vi "gyro-fitter-V1.vi"() -> ()   [LabVIEW 2018]
uses:
  plot refs -- filter related.ctl
  cursor window action.ctl
  publisher action.ctl
  circle corners.ctl
  lorentzian.ctl
  peak -- parameters -- complex fit.ctl
  wavepacket.ctl
  filter method control.ctl
  parameters -- scan monitor control.ctl
panel:
  in  "Tab :  Fit controls":T1(tab)
  out "lorentzian":T2={"A (VHz)"=1.3498083421914207e-06, "f (Hz)"=20818.316775416508, "G (Hz)"=65.7151812568016, "phi(rad)"=4.172856066514944, "Q"=316.7961554281156, "Norm  Ampl"=nan, "bg (V)"=-2.924526385728085e-08-2.2207879205523747e-08i, "4corners"={"z (-pi/2)"=-5.7420040702404924e-08-2.9278119892568764e-08i, "z(inf)"=-2.924526385728085e-08-2.2207879205523747e-08i, "z (pi/2)"=-3.6315504544325864e-08+5.9668976396003224e-09i, "z center"=-4.6867772623365394e-08-1.1655611126484221e-08i, "z(0)"=-6.449028138944994e-08-1.1033430474446945e-09i, "radius"=2.0540281809718265e-08}} {"bg (V)" format="%#9_9f"; "Q" format="%#9_9f"; "phi(rad)" format="%#9_9f"; "G (Hz)" format="%#9_9f"; "f (Hz)" format="%#9_9f"}
  in  "Plot: fragment - filter":cluster{dbl[], dbl[]}[](graph)=[{array[248 elements], array[248 elements]}, {array[248 elements], array[248 elements]}, {array[248 elements], array[248 elements]}, {array[248 elements], array[248 elements]}]
  out "Plot: phase around center":cluster{dbl[], dbl[]}[](graph)
  out "Plot: fragment":cluster{dbl[], dbl[]}[](graph)
  out "Plot: complex plane":cluster{dbl[], dbl[]}[](graph)=[{array[248 elements], array[248 elements]}, {[-2.632749081364713e-08, -2.6489457070801555e-08, -2.6972801537635557e-08, -2.7769901583171174e-08, -2.886818646352582e-08, -3.025033557005272e-08, -3.189455158568609e-08, -3.3774904241652344e-08, -3.586173925329867e-08, -3.81221459858766e-08, -4.0520476474911847e-08, -4.301890761589914e-08, -4.557803765725468e-08, -4.815750758947611e-08, -5.0716637630831656e-08, -5.321506877181894e-08, -5.561339926085419e-08, -5.7873805993432123e-08, -5.996064100507845e-08, -6.184099366104471e-08, -6.348520967667807e-08, -6.486735878320497e-08, -6.596564366355961e-08, -6.676274370909523e-08, -6.724608817592924e-08, -6.740805443308366e-08, -6.724608817592924e-08, -6.676274370909523e-08, -6.596564366355961e-08, -6.486735878320496e-08, -6.348520967667807e-08, -6.18409936610447e-08, -5.996064100507845e-08, -5.787380599343211e-08, -5.5613399260854173e-08, -5.321506877181894e-08, -5.071663763083165e-08, -4.815750758947611e-08, -4.5578037657254674e-08, -4.3018907615899126e-08, -4.052047647491185e-08, -3.81221459858766e-08, -3.586173925329867e-08, -3.377490424165234e-08, -3.1894551585686074e-08, -3.025033557005271e-08, -2.886818646352582e-08, -2.776990158317117e-08, -2.6972801537635557e-08, -2.6489457070801555e-08], [-1.1655611126484221e-08, -9.081231188950172e-09, -6.547450760891066e-09, -4.0942290732644576e-09, -1.7602548975678168e-09, 4.176635991995252e-10, 2.4051793413181066e-09, 4.1709480182503586e-09, 5.687122403141979e-09, 6.929791520224554e-09, 7.879357735187145e-09, 8.520845821576428e-09, 8.844139129063635e-09, 8.844139129063635e-09, 8.520845821576428e-09, 7.879357735187142e-09, 6.929791520224554e-09, 5.687122403141975e-09, 4.170948018250355e-09, 2.4051793413181033e-09, 4.1766359919952687e-10, -1.7602548975678184e-09, -4.0942290732644625e-09, -6.547450760891066e-09, -9.081231188950175e-09, -1.1655611126484228e-08, -1.4229991064018272e-08, -1.676377149207738e-08, -1.9216993179703993e-08, -2.1550967355400627e-08, -2.3728885852167972e-08, -2.5716401594286547e-08, -2.74821702712188e-08, -2.8998344656110424e-08, -3.0241013773193e-08, -3.1190579988155584e-08, -3.183206807454487e-08, -3.215536138203208e-08, -3.215536138203208e-08, -3.183206807454487e-08, -3.1190579988155584e-08, -3.0241013773192996e-08, -2.8998344656110417e-08, -2.7482170271218794e-08, -2.571640159428654e-08, -2.372888585216796e-08, -2.1550967355400623e-08, -1.9216993179703983e-08, -1.676377149207737e-08, -1.422999106401826e-08]}, {[-2.924526385728085e-08, -3.10075147338893e-08, -3.276976561049776e-08, -3.4532016487106214e-08, -3.629426736371467e-08, -3.805651824032312e-08, -3.981876911693158e-08, -4.158101999354003e-08, -4.334327087014848e-08, -4.510552174675694e-08, -4.6867772623365394e-08, -4.8630023499973846e-08, -5.0392274376582305e-08, -5.215452525319076e-08, -5.391677612979921e-08, -5.567902700640767e-08, -5.744127788301612e-08, -5.9203528759624574e-08, -6.096577963623303e-08, -6.272803051284148e-08], [-2.2207879205523747e-08, -2.1152652397619794e-08, -2.0097425589715843e-08, -1.904219878181189e-08, -1.7986971973907936e-08, -1.6931745166003982e-08, -1.5876518358100032e-08, -1.4821291550196078e-08, -1.3766064742292127e-08, -1.2710837934388175e-08, -1.1655611126484221e-08, -1.0600384318580269e-08, -9.545157510676317e-09, -8.489930702772363e-09, -7.434703894868411e-09, -6.379477086964459e-09, -5.324250279060506e-09, -4.269023471156552e-09, -3.2137966632526018e-09, -2.158569855348648e-09]}, {[-5.7420040702404924e-08, -5.636481389450097e-08, -5.5309587086597017e-08, -5.425436027869306e-08, -5.319913347078911e-08, -5.214390666288516e-08, -5.10886798549812e-08, -5.0033453047077255e-08, -4.89782262391733e-08, -4.792299943126935e-08, -4.6867772623365394e-08, -4.581254581546144e-08, -4.475731900755749e-08, -4.370209219965353e-08, -4.264686539174958e-08, -4.1591638583845626e-08, -4.053641177594168e-08, -3.948118496803772e-08, -3.842595816013377e-08, -3.737073135222982e-08], [-2.9278119892568764e-08, -2.751586901596031e-08, -2.5753618139351856e-08, -2.39913672627434e-08, -2.2229116386134948e-08, -2.0466865509526493e-08, -1.8704614632918037e-08, -1.6942363756309585e-08, -1.518011287970113e-08, -1.3417862003092673e-08, -1.1655611126484221e-08, -9.893360249875765e-09, -8.13110937326731e-09, -6.368858496658857e-09, -4.606607620050402e-09, -2.8443567434419492e-09, -1.0821058668334936e-09, 6.801450097749588e-10, 2.4423958863834177e-09, 4.20464676299187e-09]}, {[-0.03712059630022613, -0.04038900428695615, -0.043632170488046795, -0.04684806803019193, -0.050034687082109765, -0.053190036110621716, -0.05631214312529604, -0.05939905691087754, -0.06244884824673365, -0.06545961111255436, -0.06842946387955313, -0.07135655048642349, -0.07423904159931691, -0.07707513575511701, -0.07986306048729519, -0.08260107343364476, -0.08528746342520038, -0.08792055155566313, -0.09049869223066223, -0.09302027419619781], [0.13121393299301523, 0.1302450136134994, 0.12919469531706476, 0.12806363451845718, 0.1268525380938582, 0.12556216293911035, 0.12419331549668176, 0.12274685125166607, 0.12122367419713193, 0.11962473626915691, 0.11795103675189833, 0.11620362165307317, 0.11438358305023741, 0.11249205840827295, 0.11053022986850931, 0.10849932350992353, 0.10640060858288088, 0.10423539671589463, 0.10200504109590092, 0.09971093562256111]}, {[-0.0412038570844881, -0.04483178994975843, -0.04843170443296904, -0.05200135070475014, -0.05553849785237894, -0.059040935274027206, -0.0625064740603157, -0.06593294836231116, -0.06931821674511145, -0.07266016352617244, -0.07595670009754107, -0.07920576623116717, -0.08240533136647886, -0.08555339587941699, -0.08864799233213477, -0.09168718670258277, -0.09466907959320953, -0.09759180741802317, -0.10045354356727218, -0.10325249954901668], [0.14564746968253484, 0.1445719691712723, 0.14340611586222982, 0.1421506383757754, 0.14080632134447055, 0.1393740049227004, 0.13785458426160468, 0.13624900894963726, 0.13455828241910436, 0.13278346131905208, 0.13092565485489507, 0.12898602409519913, 0.12696578124605143, 0.12486618889347091, 0.12268855921433326, 0.12043425315630304, 0.11810467958728571, 0.11570129441493096, 0.11322559967673795, 0.11067914260133077]}, {array[248 elements], array[248 elements]}]
  in  "scale gauge: Plot: complex plane":dbl(slide)=0.00275 min=0.0 max=0.3 step=1e-06 scale=1e-05..0.5 scale format="%#_3p"
  out "Plot: phase":cluster{"omega out":dbl[], dbl[]}(graph)
  out "Plot: win omega":T4(graph)
  out "Plot: dz/domega":cluster{"omega out":dbl[], dbl[]}(graph)
  in  "Plot: complex plane - filter":cluster{dbl[], dbl[]}[](graph)=[{array[248 elements], array[248 elements]}, {array[248 elements], array[248 elements]}, {[1.0007727048625014e-06, 9.989970596885263e-07, 9.936771318268878e-07, 9.848339166024118e-07, 9.725023141455088e-07, 9.567309916573026e-07, 9.375821913424224e-07, 9.151314847674563e-07, 8.894674746145036e-07, 8.606914450068672e-07, 8.289169617868905e-07, 7.942694243234624e-07, 7.568855706179972e-07, 7.169129376620118e-07, 6.745092791760248e-07, 6.298419430276915e-07, 5.830872107862246e-07, 5.344296020195755e-07, 4.840611460799999e-07, 4.3218062425193193e-07, 3.7899278525307166e-07, 3.247075371847349e-07, 2.6953911912047683e-07, 2.1370525560234447e-07, 1.574262973815776e-07, 1.0092435179486355e-07, 4.4422406208149694e-08, -1.1856552012617152e-08, -6.76904155307497e-08, -1.228588335950076e-07, -1.7714408166334431e-07, -2.303319206622046e-07, -2.822124424902725e-07, -3.325808984298484e-07, -3.812385071964974e-07, -4.2799323943796406e-07, -4.726605755862975e-07, -5.150642340722845e-07, -5.550368670282699e-07, -5.924207207337353e-07, -6.27068258197163e-07, -6.588427414171397e-07, -6.876187710247764e-07, -7.13282781177729e-07, -7.357334877526951e-07, -7.548822880675753e-07, -7.706536105557815e-07, -7.829852130126845e-07, -7.918284282371605e-07, -7.97148356098799e-07, -7.989240012727741e-07, -7.97148356098799e-07, -7.918284282371605e-07, -7.829852130126845e-07, -7.706536105557813e-07, -7.548822880675751e-07, -7.357334877526949e-07, -7.13282781177729e-07, -6.876187710247761e-07, -6.588427414171397e-07, -6.27068258197163e-07, -5.924207207337349e-07, -5.550368670282699e-07, -5.150642340722845e-07, -4.726605755862974e-07, -4.2799323943796427e-07, -3.8123850719649685e-07, -3.3258089842984826e-07, -2.82212442490272e-07, -2.3033192066220443e-07, -1.7714408166334437e-07, -1.2285883359500722e-07, -6.769041553074954e-08, -1.185655201261657e-08, 4.442240620814987e-08, 1.0092435179486354e-07, 1.5742629738157798e-07, 2.1370525560234442e-07, 2.6953911912047736e-07, 3.247075371847351e-07, 3.7899278525307145e-07, 4.3218062425193225e-07, 4.840611460799998e-07, 5.344296020195761e-07, 5.830872107862246e-07, 6.298419430276921e-07, 6.74509279176025e-07, 7.169129376620118e-07, 7.568855706179976e-07, 7.942694243234626e-07, 8.289169617868909e-07, 8.606914450068672e-07, 8.894674746145036e-07, 9.151314847674565e-07, 9.375821913424224e-07, 9.567309916573028e-07, 9.725023141455088e-07, 9.848339166024118e-07, 9.93677131826888e-07, 9.989970596885263e-07], [-7.941413356603459e-08, -2.2912187979320604e-08, 3.336677024144617e-08, 8.920063375957865e-08, 1.4436905182383665e-07, 1.9865429989217332e-07, 2.518421388910337e-07, 3.0372266071910163e-07, 3.5409111665867737e-07, 4.027487254253263e-07, 4.4950345766679327e-07, 4.941707938151267e-07, 5.365744523011137e-07, 5.76547085257099e-07, 6.139309389625643e-07, 6.485784764259922e-07, 6.803529596459688e-07, 7.091289892536055e-07, 7.347929994065581e-07, 7.572437059815242e-07, 7.763925062964043e-07, 7.921638287846105e-07, 8.044954312415137e-07, 8.133386464659896e-07, 8.186585743276281e-07, 8.204342195016031e-07, 8.186585743276281e-07, 8.133386464659896e-07, 8.044954312415136e-07, 7.921638287846105e-07, 7.763925062964043e-07, 7.572437059815242e-07, 7.347929994065581e-07, 7.091289892536053e-07, 6.803529596459686e-07, 6.485784764259922e-07, 6.139309389625643e-07, 5.765470852570989e-07, 5.365744523011135e-07, 4.941707938151265e-07, 4.495034576667934e-07, 4.027487254253263e-07, 3.540911166586773e-07, 3.037226607191014e-07, 2.518421388910335e-07, 1.9865429989217305e-07, 1.4436905182383667e-07, 8.920063375957859e-08, 3.3366770241446023e-08, -2.2912187979320816e-08, -7.941413356603488e-08, -1.3591607915274855e-07, -1.921950373735154e-07, -2.4802890089164793e-07, -3.0319731895590604e-07, -3.5748256702424276e-07, -4.106704060231032e-07, -4.6255092785117075e-07, -5.129193837907467e-07, -5.615769925573957e-07, -6.083317247988627e-07, -6.529990609471961e-07, -6.954027194331829e-07, -7.353753523891683e-07, -7.727592060946336e-07, -8.074067435580613e-07, -8.391812267780381e-07, -8.679572563856746e-07, -8.936212665386275e-07, -9.160719731135933e-07, -9.352207734284734e-07, -9.509920959166797e-07, -9.633236983735828e-07, -9.72166913598059e-07, -9.774868414596972e-07, -9.792624866336723e-07, -9.774868414596972e-07, -9.721669135980588e-07, -9.633236983735828e-07, -9.509920959166796e-07, -9.352207734284736e-07, -9.160719731135932e-07, -8.936212665386273e-07, -8.679572563856744e-07, -8.391812267780379e-07, -8.07406743558061e-07, -7.727592060946332e-07, -7.353753523891682e-07, -6.954027194331825e-07, -6.529990609471957e-07, -6.083317247988619e-07, -5.615769925573952e-07, -5.129193837907467e-07, -4.6255092785117033e-07, -4.1067040602310277e-07, -3.574825670242419e-07, -3.0319731895590556e-07, -2.480289008916479e-07, -1.921950373735149e-07, -1.3591607915274848e-07]}, {[8.158298491348722e-07, 1.4464037823280978e-07, -1.4742601783239322e-07], [2.2455224868565569e-07, -4.250242519508206e-08, -2.2568975850353674e-07]}, {[1.4646634674448616e-08, 5.3243073422403955e-09, -3.998019989967825e-09, -1.3320347322176047e-08, -2.2642674654384265e-08, -3.1965001986592484e-08, -4.128732931880071e-08, -5.060965665100893e-08, -5.993198398321715e-08, -6.925431131542536e-08, -7.857663864763358e-08, -8.78989659798418e-08, -9.722129331205003e-08, -1.0654362064425824e-07, -1.1586594797646647e-07, -1.2518827530867468e-07, -1.345106026408829e-07, -1.4383292997309114e-07, -1.5315525730529934e-07, -1.6247758463750758e-07], [3.0693237684966145e-08, 2.3232631101344026e-08, 1.5772024517721908e-08, 8.31141793409979e-09, 8.508113504776711e-10, -6.609795233144444e-09, -1.4070401816766566e-08, -2.1531008400388688e-08, -2.8991614984010803e-08, -3.645222156763292e-08, -4.391282815125503e-08, -5.137343473487716e-08, -5.8834041318499277e-08, -6.629464790212139e-08, -7.375525448574352e-08, -8.121586106936564e-08, -8.867646765298775e-08, -9.613707423660988e-08, -1.0359768082023198e-07, -1.1105828740385411e-07]}, {[1.4464037823280976e-07, 1.5714332117450805e-07, 1.6964626411620634e-07, 1.8214920705790464e-07, 1.9465214999960293e-07, 2.0715509294130122e-07, 2.1965803588299952e-07, 2.321609788246978e-07, 2.446639217663961e-07, 2.5716686470809437e-07, 2.696698076497927e-07, 2.82172750591491e-07, 2.946756935331893e-07, 3.0717863647488754e-07, 3.1968157941658586e-07, 3.321845223582842e-07, 3.4468746529998245e-07, 3.571904082416807e-07, 3.6969335118337904e-07, 3.8219629412507736e-07], [-4.250242519508206e-08, -4.250242519508206e-08, -4.250242519508206e-08, -4.250242519508206e-08, -4.250242519508206e-08, -4.250242519508206e-08, -4.250242519508206e-08, -4.250242519508206e-08, -4.250242519508206e-08, -4.250242519508206e-08, -4.250242519508206e-08, -4.250242519508206e-08, -4.250242519508206e-08, -4.250242519508206e-08, -4.250242519508206e-08, -4.250242519508206e-08, -4.250242519508206e-08, -4.250242519508206e-08, -4.250242519508206e-08, -4.250242519508206e-08]}]
  in  "scale gauge: Plot: complex plane - filter":dbl(slide)=0.000254 min=0.0 max=0.3 step=1e-06 scale=1e-05..0.5 scale format="%#_5g"
  in  "scan monitor control":T5={"gamma acc. frac. - min "=0.3, "gamma acc frac.. - max"=3.0, "peak acc. fraction (af)"=5.0, "min peak acc. window (kHz)"=0.5, "use"=enum."fraction", "abs gamma min(kHz)"=0.005, "abs gamma max(kHz)"=5.0, "# points"=5, "gamma-factor (fa)"=3.0, "interpolate"=enum."line", "init"=TRUE, "Unique strike parameters"=TRUE, "max peak acc. window (kHz)"=10.0, "spacing factor"=1.5, "iterate #"=1, "overwrite ctl?"=FALSE, "write _m files?"=FALSE, "max slope (kHz/sweep)"=0.5, "funnel state"=enum."funnel open"}
  in  "parameters -- scan monitor control.ctlparameters: complex fit":T6={"main VI path"=path "", "scale factor"=3.0, "# of grid points"=200, "parameters: wavepacket"={"R"=0.5, "wave number"=22.0, "delta k"=7.0, "radii vector"=[], "radial section"=[], "wave vector"=22.0, "wavepacket is"=TRUE}, "span"=0.27789, "interference ?"=enum."cp z center", "filter method"=enum."three"} {"span" min=0.0 max=0.5 step=1e-05 scale=0.0001..0.5 scale format="%#_5f"; "parameters: wavepacket"."delta k" format="%#_3f"; "parameters: wavepacket"."wave number" format="%#_3f"; "parameters: wavepacket"."R" format="%#_3f"}
  in  "Tab :  Fit controls 2":enum32{"complex plane"}(tab)
  in  "plot staff!":enum16{"plot", "do not plot", "a"}(ring)
  in  "use fast fit!":bool
  out "# of points":dbl=953.475933538175
  out "win center (kHz)":dbl=3399.029286744401
  out "win width (kHz)":dbl=76.27809365793496
  # "three strikes"
  # "search window"
  # "linear extrapolation"
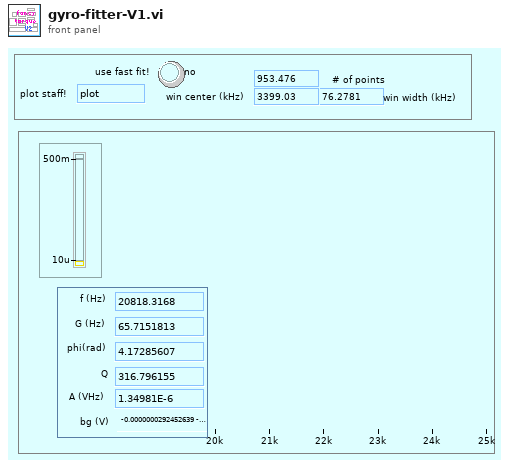
[diagram p1: front panel]
types:
  T1 = enum32{"complex plane", "complex plane 3", "complex plane 4"}
  T2 = typedef "lorentzian.ctl" = cluster{"A (VHz)":dbl, "f (Hz)":dbl, "G (Hz)":dbl, "phi(rad)":dbl, "Q":dbl, "Norm  Ampl":dbl, "bg (V)":cdb, "4corners":T3}
  T3 = typedef "circle corners.ctl" = cluster{"z (-pi/2)":cdb, "z(inf)":cdb, "z (pi/2)":cdb, "z center":cdb, "z(0)":cdb, "radius":dbl}
  T4 = cluster{"omega out":dbl[], "win omega out":dbl[]}
  T5 = typedef "parameters -- scan monitor control.ctl" = cluster{"gamma acc. frac. - min ":dbl, "gamma acc frac.. - max":dbl, "peak acc. fraction (af)":dbl, "min peak acc. window (kHz)":dbl, "use":enum16{"window", "fraction"}, "abs gamma min(kHz)":dbl, "abs gamma max(kHz)":dbl, "# points":i32, "gamma-factor (fa)":dbl, "interpolate":enum16{"line", "last"}, "init":bool, "Unique strike parameters":bool, "max peak acc. window (kHz)":dbl, "spacing factor":dbl, "iterate #":i32, "overwrite ctl?":bool, "write _m files?":bool, "max slope (kHz/sweep)":dbl, "funnel state":enum16{"funnel open", "funnel closed"}}
  T6 = typedef "peak -- parameters -- complex fit.ctl" = cluster{"main VI path":path, "scale factor":dbl, "# of grid points":i32, "parameters: wavepacket":T7, "span":dbl, "interference ?":enum16{"cp z center", "pm zcenter", "fancy"}, "filter method":T8}
  T7 = typedef "wavepacket.ctl" = cluster{"R":dbl, "wave number":dbl, "delta k":dbl, "radii vector":dbl[], "radial section":cdb[], "wave vector":dbl, "wavepacket is":bool}
  T8 = typedef "filter method control.ctl" = enum16{"four", "five", "one", "two", "three", "zero", "minus one", "minus two"}
  T9 = typedef "publisher action.ctl" = enum16{"set", "get", "init", "check"}
  T10 = typedef "plot refs -- filter related.ctl" = cluster{"Plot: complex plane - filter":refnum<vi>, "Plot: dz/domega":refnum<vi>, "Plot: fragment filter":refnum<vi>, "Plot: win omega":refnum<vi>, "Plot: phase":refnum<vi>, "Plot: phase around center":refnum<vi>, "Plot: complex plane":refnum<vi>, "Plot: fragment":refnum<vi>}
  T11 = typedef "cursor window action.ctl" = enum16{"balance", "h. offset change", "cursor moves", "change center", "change window", "init", "check", "reset", "set y to middle", "idle", "-write all Y", "-write left.X", "-write center.X", "-write right.X", "-write all X", "-change center", "-change window", "-change skew", "-read cursor 2", "-read cursor 1", "-read cursor 0", "-read all cursors", "-reset", "-read plot scale", "-set y to middle", "-Q: center.Y is visible", "-Q: window is visible", "-parse center.Y", "-right left from center", "-left move", "-right move", "-set center.Y", "-empty", "-set cursors to default", "-check", "-write center.Y", "-copy cursor 1", "-copy cursor 0", "-copy cursor 2", "move right", "move left", "shrink", "broaden", "skew up", "skew down", "-write plot scale", "zoom X", "change cen&win", "zoom to all data", "color--red", "color--green", "color--yellow", "read", "zoom out", "zoom in", "slide right", "slide left", "set range aspect ratio to 1"}
  T12 = typedef "cursor winow.ctl" = cluster{"left":dbl, "right ":dbl, "center":dbl, "window":dbl, "cursors":i32[], "relative":i32, "absolute":i32, "fixed vertical offset":dbl, "vertical offset":dbl, "skew":dbl, "default window frac":dbl, "kind":enum16{"symmetric", "skewed", "fancy"}, "skew.left":dbl, "skew.right":dbl, "Plot ref":refnum<vi>, "wing order":enum16{"forw", "back"}}
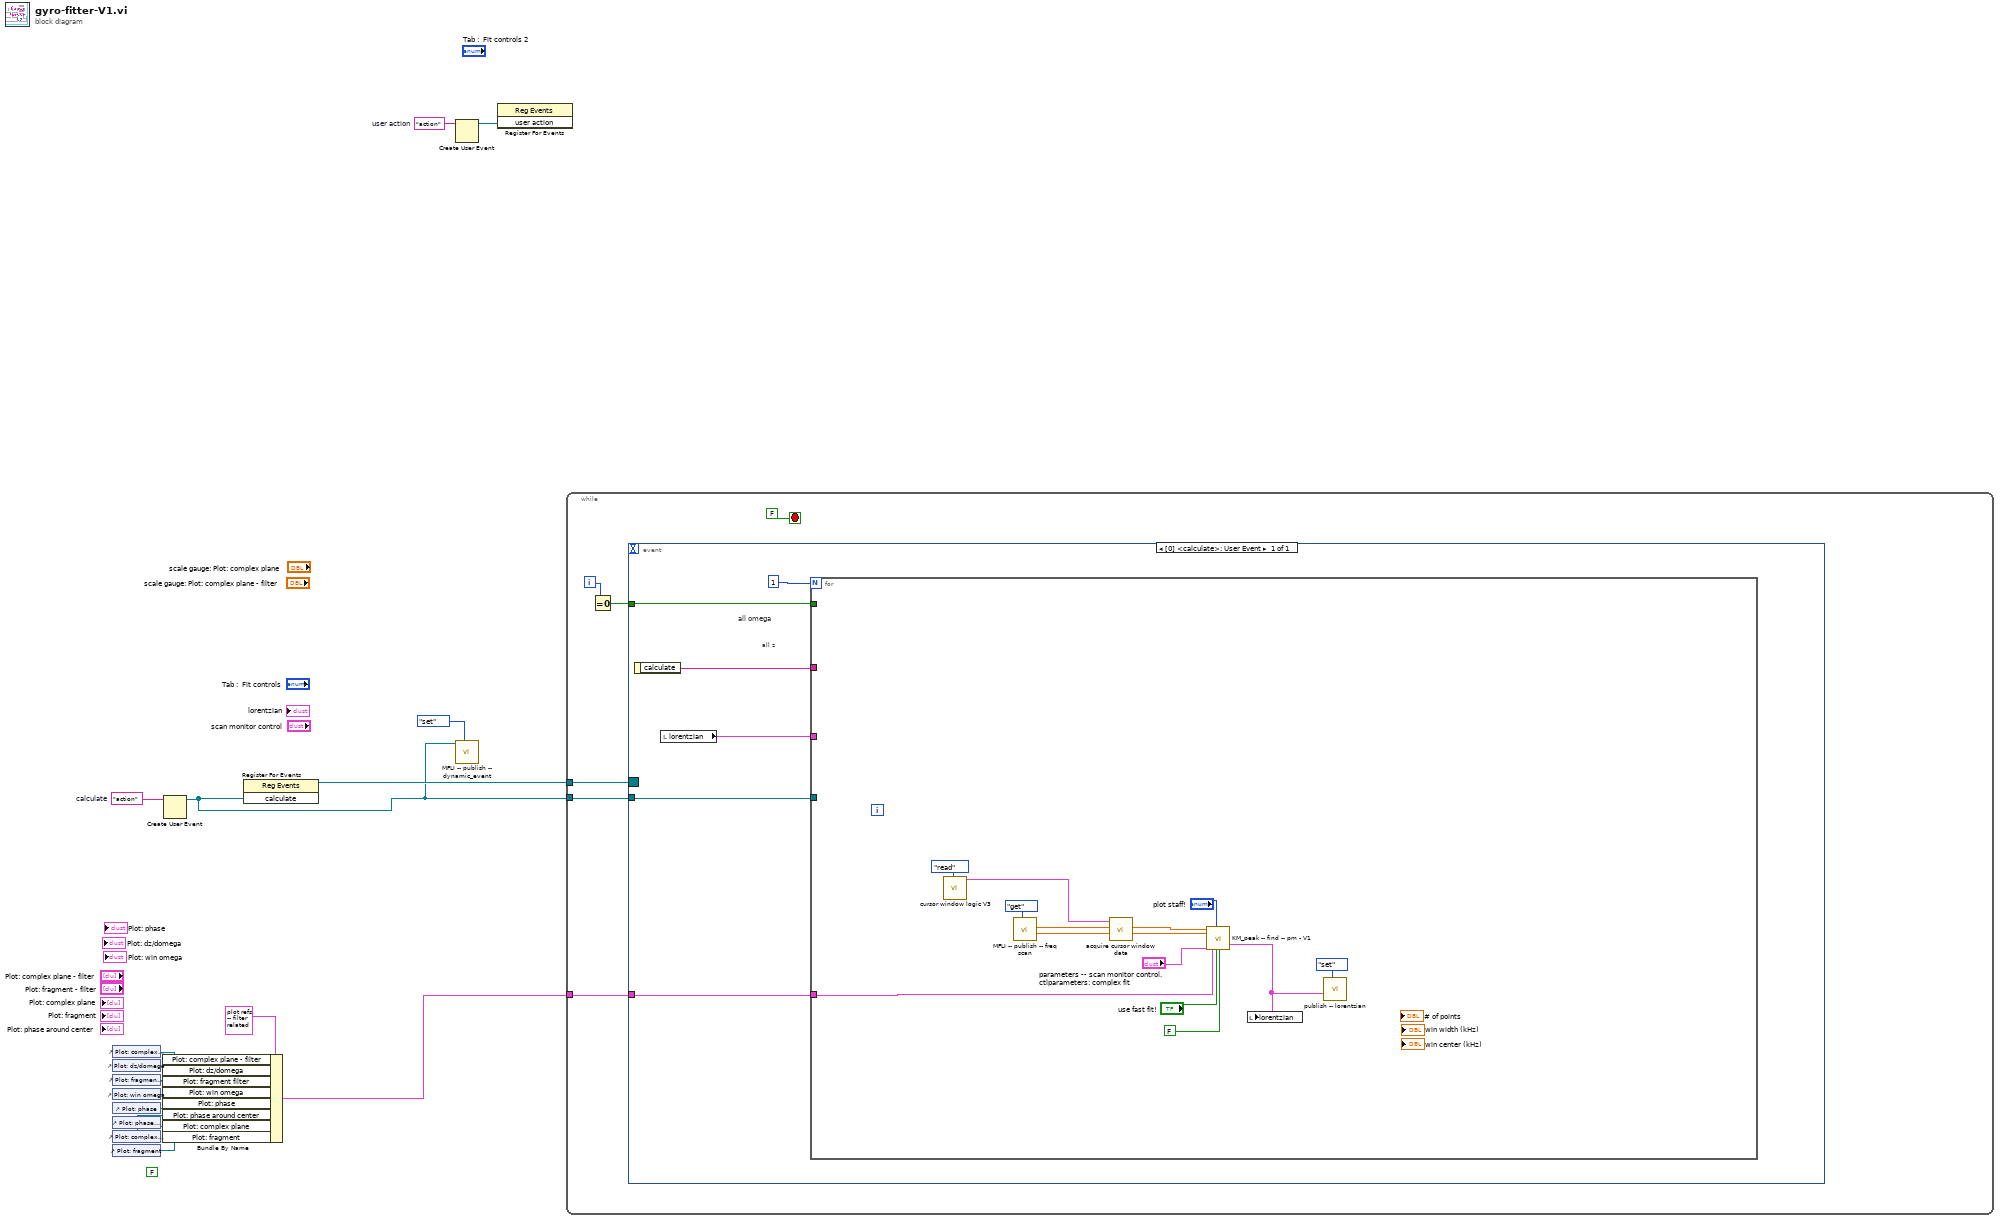
[diagram p0: block diagram]
diagram:
  w14 = "action"  # user action
  w15 = "action"  # calculate
  (unwired) FALSE
  n1 = control-ref of="Plot: complex plane - filter"() -> (w11:refnum<vi>)
  n2 = control-ref of="Plot: dz/domega"() -> (w10:refnum<vi>)
  n3 = control-ref of="Plot: fragment - filter"() -> (w9:refnum<vi>)
  n4 = control-ref of="Plot: win omega"() -> (w8:refnum<vi>)
  n5 = control-ref of="Plot: phase"() -> (w7:refnum<vi>)
  n6 = control-ref of="Plot: phase around center"() -> (w5:refnum<vi>)
  n7 = control-ref of="Plot: complex plane"() -> (w4:refnum<vi>)
  n8 = control-ref of="Plot: fragment"() -> (w3:refnum<vi>)
  n9 = Bundle By Name(cluster=T10 {"Plot: complex plane - filter"=refnum, "Plot: dz/domega"=refnum, "Plot: fragment filter"=refnum, "Plot: win omega"=refnum, "Plot: phase"=refnum, "Plot: phase around center"=refnum, "Plot: complex plane"=refnum, "Plot: fragment"=refnum} ("plots: filter related"), "Plot: complex plane - filter"=w11, "Plot: dz/domega"=w10, "Plot: fragment filter"=w9, "Plot: win omega"=w8, "Plot: phase"=w7, "Plot: phase around center"=w5, "Plot: complex plane"=w4, "Plot: fragment"=w3) -> (w6:T10)
  n10 = Create User Event(user event datatype=w15) -> (user event=w2:refnum<user-event>)  [unwired: 1 in, 1 out]
  n11 = register-events(w2) -> (reference out=w16:refnum<event-registration>)  [unwired: 2 in, 1 out]
  n12 = Create User Event(user event datatype=w14) -> (user event=w13:refnum<user-event>)  [unwired: 1 in, 1 out]
  n13 = call "MFLI -- publish -- dynamic_event.vi"("publisher action"=publisher_action."set", "dynamic event"=w2) -> ()  [unwired: 9 in, 1 out]
  n14 = register-events(w13) -> ()  [unwired: 2 in, 2 out]
  n15 = while {
    tunnel: w16 -> [w22]
    tunnel: w2 -> [w20]
    tunnel: w6 -> [w18]
    i -> [w19]
    stop <- FALSE stop-if-true
    n16 = Equal To 0?(x=w19) -> (x = 0?=w17:bool)
    n17 = event shown="[0] <calculate>: User Event" {
      selector: w22 -> [_]
      dyn-events: _ -> [_]
      timeout: _ -> [_]
      tunnel: w20 -> [w27]
      tunnel: w18 -> [w25]
      tunnel: w17 -> [w24]
      event User Event {
        # "all z"
        # "all omega"
        n18 = event-data() -> ("calculate"=w28:string)  [unwired: 1 in]
        n19 = local read "lorentzian"() -> (w23:T2)
        n20 = for {
          N: 1 -> [_]
          tunnel: w28 -> [_]
          tunnel: w27 -> [_]
          tunnel: w25 -> [w42]
          tunnel: w24 -> [_]
          tunnel: w23 -> [_]
          n21 = call "cursor window logic V3.vi"("cursor window action"=cursor_window_action."read") -> ("cursor window out"=w34:T12)  [unwired: 9 in, 1 out]
          n22 = call "MFLI -- publish -- freq scan.vi"("publisher action"=publisher_action."get") -> ("Voltage out (V)"=w29:cdb[], "Freq out (Hz)"=w30:dbl[])  [unwired: 9 in]
          n23 = call "acquire cursor window data.vi"("z in"=w29, "omega in"=w30, "cursor window"=w34) -> ("z out"=w35:cdb[], "omega  out"=w36:dbl[])  [unwired: 4 in, 3 out]
          n24 = call "KM_peak -- find -- pm - V1.vi"("omega in"=w36, "z in"=w35, "parameters: complex fit"="parameters -- scan monitor control.ctlparameters: complex fit", "plots: filter related"=w42, "plot staff ?"="plot staff!", "just guess?"="use fast fit!", "subtract linear BG"=FALSE) -> ("pm lorentzian"=w32:T2)  [unwired: 10 in, 2 out]
          n25 = local write "lorentzian"(w32) -> ()
          n26 = call "publish -- lorentzian.vi"("publisher action"=publisher_action."set", "lorentzian IN"=w32) -> ()  [unwired: 9 in, 1 out]
        }
      }
    }
  }
